vi "MPPTracker.vi"(0 "VMPP (V)":sgl, 1 "Device Code":i32=21, 2 "ID":i32=1, 3 "Channel":u8(ring) items=["1", "2", "3", "4", "5", "6", "7", "8", "9", "10", "11", "12", "13", "14", "15", "16"], 4 "instance":i32, 5 "JV after\nevery (min)":dbl=15.0 caption="Time Target (s)", 7 "Step (V)":sgl=0.01, 8 "device area (cm2)":dbl=0.16 caption="Time Target (s)", 9 "time to check (s)":sgl=10.0, 11 "error in (no error)":errorcluster, 12 "start time":timestamp, 13 "Average over":i32, 14 "AgingFile":path=path "C:/EC-Lab Development Package/Examples/Labview/V12/DefaultAging") -> (15 "error out":errorcluster)   [LabVIEW 2020]
uses:
  base_xml.llb/Type Descriptor Enumeration__ogtk.ctl
  ActiveArray.vi
  <vilib>/Utility/file.llb/Write Delimited Spreadsheet (DBL).vi
  IntensityTemperature.vi
panel:
  out "MPP start time":timestamp
  out "Time has Elapsed":bool
  out "Data 100":dbl[][](array[numeric]) format="%.2f"
  out "finished":bool
  out "XY Graph 2":cluster{"Data 101":sgl[], "Data 101":dbl[]}(graph) caption="XY Graph"
  out "Number\nof points":i32=255
  in  "Current measurement":enum16{"P(t)", "Ewe(t)", "I(t)"}(ring) caption="Draw"
  out "time (s)":sgl
  out "V (V)":sgl
  out "J (mA/cm2)":sgl
  out "P (mW/cm2)":sgl
  out "Aging Data":sgl[][](array[numeric])
  out "<P> mW/cm2":sgl=0.01
  out "last time":i32
  in  "stop 4":bool
  in  "Average last %":dbl(slide)=25.25252525252525
  in  "starting time offset (h)":dbl
  out "CAData":sgl[][](array[numeric])=[[0.0, -0.00011507986, 2.9229916e-06, 1.0], [0.010008001, -0.00048330438, 2.9229916e-06, 1.0], [0.020016002, -0.00048330438, 2.9229916e-06, 1.0], [0.030024001, -0.0007121685, 6.7342776e-06, 1.0], [0.040032003, -0.0007121685, 3.6852487e-06, 1.0], [0.050040003, -0.00063588045, 6.362202e-07, 1.0], [0.060048003, -0.00048330438, 5.2097635e-06, 1.0], [0.070056, -0.0004070163, 2.1607345e-06, 1.0], [0.080064006, -0.00017815214, 3.6852487e-06, 1.0], [0.090072006, -0.0004070163, 3.6852487e-06, 1.0], [0.100080006, -0.0004070163, 2.1607345e-06, 1.0], [0.110088006, -0.00063588045, 2.9229916e-06, 1.0], [0.120096005, -0.0005595924, 2.9229916e-06, 1.0], [0.130104, -0.0007121685, 5.2097635e-06, 1.0], [0.140112, -0.00033072825, 5.2097635e-06, 1.0], [0.15012, -0.00063588045, 2.9229916e-06, 1.0], [0.16012801, -0.0007884566, 1.3984774e-06, 1.0], [0.170136, -0.0004070163, 5.2097635e-06, 1.0], [0.18014401, -0.00063588045, 3.6852487e-06, 1.0], [0.190152, -0.00063588045, 5.97202e-06, 1.0], [0.20016001, -0.0007121685, 5.2097635e-06, 1.0], [0.210168, -0.00033072825, 2.9229916e-06, 1.0], [0.22017601, -0.0007121685, 1.3984774e-06, 1.0], [0.230184, -0.00063588045, 5.97202e-06, 1.0], [0.24019201, -0.0007884566, 5.97202e-06, 1.0], [0.2502, -0.00063588045, 4.447506e-06, 1.0], [0.260208, -0.00063588045, 4.447506e-06, 1.0], [0.27021602, -0.0007884566, 3.6852487e-06, 1.0], [0.280224, -0.00025444018, 2.9229916e-06, 1.0], [0.290232, -0.00063588045, 4.447506e-06, 1.0], [0.30024, -0.0007884566, 5.2097635e-06, 1.0], [0.31024802, -0.00048330438, 2.9229916e-06, 1.0], [0.32025602, -0.00063588045, 2.1607345e-06, 1.0], [0.330264, -0.00063588045, 3.6852487e-06, 1.0], [0.340272, -0.00063588045, 2.9229916e-06, 1.0], [0.35028002, -0.00017815214, 5.2097635e-06, 1.0], [0.36028802, -0.0007884566, 5.97202e-06, 1.0], [0.370296, -0.00063588045, 2.9229916e-06, 1.0], [0.380304, -0.00086474465, 6.7342776e-06, 1.0], [0.39031202, -0.0004070163, 2.9229916e-06, 1.0], [0.40032002, -0.0007884566, 6.362202e-07, 1.0], [0.410328, -0.0007121685, 2.1607345e-06, 1.0], [0.420336, -0.0007884566, 6.7342776e-06, 1.0], [0.43034402, -0.00063588045, 1.3984774e-06, 1.0], [0.44035202, -0.00063588045, 2.9229916e-06, 1.0], [0.45036003, -0.00063588045, 2.1607345e-06, 1.0], [0.460368, -0.00048330438, 4.447506e-06, 1.0], [0.470376, -0.00048330438, 4.447506e-06, 1.0], [0.48038402, -0.0004070163, 2.9229916e-06, 1.0], [0.49039203, -0.00033072825, 5.2097635e-06, 1.0], [0.5004, -0.00048330438, 5.2097635e-06, 1.0], [0.51040804, -0.0005595924, 5.2097635e-06, 1.0], [0.520416, -0.0005595924, 5.97202e-06, 1.0], [0.530424, -0.0007121685, 5.2097635e-06, 1.0], [0.54043204, -0.0004070163, 2.9229916e-06, 1.0], [0.55044, -0.00025444018, 5.2097635e-06, 1.0], [0.560448, -0.00048330438, 2.9229916e-06, 1.0], [0.570456, -0.0004070163, 4.447506e-06, 1.0], [0.580464, -0.0004070163, 2.9229916e-06, 1.0], [0.59047204, -0.00063588045, 2.1607345e-06, 1.0], [0.60048, -0.0007884566, 2.1607345e-06, 1.0], [0.610488, -0.00048330438, 5.2097635e-06, 1.0], [0.62049603, -0.0004070163, 2.9229916e-06, 1.0], [0.630504, -0.0007884566, 3.6852487e-06, 1.0], [0.64051205, -0.0007884566, 2.9229916e-06, 1.0], [0.65052, -0.0005595924, 5.97202e-06, 1.0], [0.660528, -0.00048330438, 2.9229916e-06, 1.0], [0.67053604, -0.00063588045, 4.447506e-06, 1.0], [0.680544, -0.00086474465, 4.447506e-06, 1.0], [0.690552, -0.00063588045, 3.6852487e-06, 1.0], [0.70056003, -0.00063588045, 1.3984774e-06, 1.0], [0.710568, -0.0005595924, 4.447506e-06, 1.0], [0.72057605, -0.00048330438, 2.9229916e-06, 1.0], [0.730584, -0.00048330438, 3.6852487e-06, 1.0], [0.740592, -0.0007884566, 4.447506e-06, 1.0], [0.75060004, -0.0005595924, 3.6852487e-06, 1.0], [0.760608, -0.0005595924, 2.9229916e-06, 1.0], [0.77061605, -0.0007884566, 4.447506e-06, 1.0], [0.78062403, -0.0010173208, 2.1607345e-06, 1.0], [0.790632, -0.00063588045, 2.1607345e-06, 1.0], [0.80064005, -0.00025444018, 2.9229916e-06, 1.0], [0.810648, -0.0005595924, 3.6852487e-06, 1.0], [0.820656, -0.00017815214, 3.6852487e-06, 1.0], [0.83066404, -0.0005595924, 4.447506e-06, 1.0], [0.840672, -0.0005595924, 1.3984774e-06, 1.0], [0.85068005, -0.00063588045, 5.2097635e-06, 1.0], [0.86068803, -0.0007884566, 5.97202e-06, 1.0], [0.870696, -0.0004070163, 4.447506e-06, 1.0], [0.88070405, -0.00033072825, 4.447506e-06, 1.0], [0.890712, -0.0005595924, 3.6852487e-06, 1.0], [0.90072006, -0.0005595924, 4.447506e-06, 1.0], [0.91072804, -0.0007121685, 4.447506e-06, 1.0], [0.920736, -0.00063588045, 2.1607345e-06, 1.0], [0.93074405, -0.0005595924, 5.2097635e-06, 1.0], [0.940752, -0.0004070163, 2.1607345e-06, 1.0], [0.95076, -0.0004070163, 2.1607345e-06, 1.0], [0.96076804, -0.00025444018, 2.9229916e-06, 1.0], [0.970776, -0.00063588045, 3.6852487e-06, 1.0], [0.98078406, -0.00063588045, 2.9229916e-06, 1.0], [0.99079204, 0.0001270001, 2.1607345e-06, 1.0], [1.0008, 0.09945406, 5.5518736e-05, 1.0], [1.010808, 0.09960663, 2.3503935e-05, 1.0], [1.0208161, 0.09945406, 2.2741679e-05, 1.0], [1.0308241, 0.099759206, 2.5790707e-05, 1.0], [1.040832, 0.09930148, 2.4266194e-05, 1.0], [1.05084, 0.099377766, 2.1217164e-05, 1.0], [1.060848, 0.09945406, 2.2741679e-05, 1.0], [1.0708561, 0.09953035, 2.1217164e-05, 1.0], [1.0808641, 0.09953035, 2.3503935e-05, 1.0], [1.090872, 0.09953035, 2.3503935e-05, 1.0], [1.10088, 0.09968292, 2.4266194e-05, 1.0], [1.110888, 0.09945406, 2.4266194e-05, 1.0], [1.120896, 0.09953035, 2.6552963e-05, 1.0], [1.1309041, 0.099377766, 2.6552963e-05, 1.0], [1.140912, 0.09953035, 2.502845e-05, 1.0], [1.15092, 0.09922519, 2.1217164e-05, 1.0], [1.160928, 0.09953035, 2.3503935e-05, 1.0], [1.170936, 0.099377766, 1.969265e-05, 1.0], [1.1809441, 0.09930148, 2.4266194e-05, 1.0], [1.1909521, 0.09953035, 2.4266194e-05, 1.0], [1.20096, 0.09953035, 2.3503935e-05, 1.0], [1.210968, 0.09953035, 2.4266194e-05, 1.0], [1.220976, 0.09968292, 2.2741679e-05, 1.0], [1.2309841, 0.09960663, 2.4266194e-05, 1.0], [1.2409921, 0.0998355, 2.4266194e-05, 1.0], [1.251, 0.09945406, 2.1217164e-05, 1.0], [1.261008, 0.09968292, 2.502845e-05, 1.0], [1.271016, 0.09930148, 2.4266194e-05, 1.0], [1.2810241, 0.09968292, 1.8930392e-05, 1.0], [1.2910321, 0.09930148, 2.4266194e-05, 1.0], [1.30104, 0.09930148, 2.5790707e-05, 1.0], [1.311048, 0.09907261, 2.4266194e-05, 1.0], [1.321056, 0.09945406, 2.1217164e-05, 1.0], [1.3310641, 0.09968292, 2.5790707e-05, 1.0], [1.3410721, 0.09914891, 2.1979422e-05, 1.0], [1.3510801, 0.09945406, 2.502845e-05, 1.0], [1.361088, 0.09945406, 2.5790707e-05, 1.0], [1.371096, 0.09960663, 2.1217164e-05, 1.0], [1.381104, 0.09930148, 2.4266194e-05, 1.0], [1.3911121, 0.09930148, 2.4266194e-05, 1.0], [1.4011201, 0.09998807, 2.4266194e-05, 1.0], [1.411128, 0.09968292, 2.4266194e-05, 1.0], [1.421136, 0.09960663, 2.1217164e-05, 1.0], [1.431144, 0.09998807, 2.3503935e-05, 1.0], [1.4411521, 0.09968292, 2.1217164e-05, 1.0], [1.4511601, 0.09953035, 2.5790707e-05, 1.0], [1.461168, 0.09960663, 2.5790707e-05, 1.0], [1.471176, 0.09968292, 2.2741679e-05, 1.0], [1.481184, 0.09930148, 2.4266194e-05, 1.0], [1.4911921, 0.09945406, 2.2741679e-05, 1.0], [1.5012001, 0.09960663, 2.0454907e-05, 1.0], [1.511208, 0.09945406, 2.3503935e-05, 1.0], [1.521216, 0.099377766, 1.969265e-05, 1.0], [1.531224, 0.09930148, 2.1217164e-05, 1.0], [1.5412321, 0.09914891, 2.2741679e-05, 1.0], [1.5512401, 0.09953035, 2.2741679e-05, 1.0], [1.5612481, 0.099377766, 2.2741679e-05, 1.0], [1.571256, 0.099377766, 2.5790707e-05, 1.0], [1.581264, 0.099759206, 2.4266194e-05, 1.0], [1.5912721, 0.09968292, 2.2741679e-05, 1.0], [1.6012801, 0.09930148, 2.4266194e-05, 1.0], [1.6112881, 0.09930148, 2.4266194e-05, 1.0], [1.621296, 0.09960663, 2.1217164e-05, 1.0], [1.631304, 0.09968292, 2.5790707e-05, 1.0], [1.641312, 0.09953035, 2.5790707e-05, 1.0], [1.6513201, 0.09930148, 2.502845e-05, 1.0], [1.6613281, 0.09945406, 2.4266194e-05, 1.0], [1.671336, 0.09953035, 2.1217164e-05, 1.0], [1.681344, 0.099377766, 2.4266194e-05, 1.0], [1.691352, 0.09960663, 2.2741679e-05, 1.0], [1.7013601, 0.09968292, 2.3503935e-05, 1.0], [1.7113681, 0.09907261, 2.5790707e-05, 1.0], [1.7213761, 0.09953035, 2.4266194e-05, 1.0], [1.731384, 0.099377766, 2.2741679e-05, 1.0], [1.741392, 0.09960663, 2.502845e-05, 1.0], [1.7514001, 0.09953035, 2.502845e-05, 1.0], [1.7614081, 0.09945406, 2.6552963e-05, 1.0], [1.7714161, 0.099377766, 2.502845e-05, 1.0], [1.781424, 0.09960663, 2.5790707e-05, 1.0], [1.791432, 0.09907261, 2.502845e-05, 1.0], [1.8014401, 0.09930148, 2.0454907e-05, 1.0], [1.8114481, 0.09968292, 2.1979422e-05, 1.0], [1.8214561, 0.09930148, 2.2741679e-05, 1.0], [1.831464, 0.09930148, 2.4266194e-05, 1.0], [1.841472, 0.09914891, 2.0454907e-05, 1.0], [1.85148, 0.099377766, 2.2741679e-05, 1.0], [1.8614881, 0.09953035, 2.502845e-05, 1.0], [1.8714961, 0.09945406, 2.3503935e-05, 1.0], [1.881504, 0.09907261, 2.502845e-05, 1.0], [1.891512, 0.099377766, 2.2741679e-05, 1.0], [1.90152, 0.09945406, 2.5790707e-05, 1.0], [1.9115281, 0.09953035, 2.5790707e-05, 1.0], [1.9215361, 0.099759206, 2.4266194e-05, 1.0], [1.9315441, 0.09945406, 2.6552963e-05, 1.0], [1.941552, 0.09945406, 2.0454907e-05, 1.0], [1.95156, 0.09945406, 2.5790707e-05, 1.0], [1.9615681, 0.09991179, 2.5790707e-05, 1.0], [1.9715761, 0.09945406, 2.3503935e-05, 1.0], [1.9815841, 0.09930148, 2.3503935e-05, 1.0], [1.991592, 0.09960663, 2.5790707e-05, 1.0], [2.0016, 0.19969657, 6.3903564e-05, 1.0], [2.0116081, 0.19939142, 4.256037e-05, 1.0], [2.021616, 0.19931513, 4.408488e-05, 1.0], [2.031624, 0.1994677, 4.332262e-05, 1.0], [2.0416322, 0.199544, 4.332262e-05, 1.0], [2.05164, 0.1994677, 4.4847136e-05, 1.0], [2.0616481, 0.19962028, 4.332262e-05, 1.0], [2.071656, 0.19977286, 4.332262e-05, 1.0], [2.081664, 0.19992544, 4.256037e-05, 1.0], [2.0916722, 0.19977286, 4.4847136e-05, 1.0], [2.10168, 0.19977286, 4.408488e-05, 1.0], [2.1116881, 0.20007801, 4.4847136e-05, 1.0], [2.121696, 0.19992544, 4.103585e-05, 1.0], [2.131704, 0.199544, 4.256037e-05, 1.0], [2.1417122, 0.199544, 4.6371653e-05, 1.0], [2.15172, 0.19969657, 4.256037e-05, 1.0], [2.1617281, 0.199544, 4.256037e-05, 1.0], [2.171736, 0.19984914, 4.256037e-05, 1.0], [2.181744, 0.1994677, 4.256037e-05, 1.0], [2.1917522, 0.20000172, 4.256037e-05, 1.0], [2.20176, 0.199544, 4.6371653e-05, 1.0], [2.2117682, 0.1994677, 4.0273593e-05, 1.0], [2.221776, 0.19969657, 4.332262e-05, 1.0], [2.231784, 0.19962028, 4.332262e-05, 1.0], [2.241792, 0.199544, 4.408488e-05, 1.0], [2.2518, 0.19977286, 4.332262e-05, 1.0], [2.2618082, 0.1994677, 4.408488e-05, 1.0], [2.271816, 0.19969657, 4.6371653e-05, 1.0], [2.281824, 0.19969657, 4.408488e-05, 1.0], [2.291832, 0.1994677, 4.332262e-05, 1.0], [2.30184, 0.19984914, 4.408488e-05, 1.0], [2.3118482, 0.19923884, 3.9511335e-05, 1.0], [2.321856, 0.19962028, 4.256037e-05, 1.0], [2.331864, 0.19969657, 4.1798106e-05, 1.0], [2.341872, 0.19969657, 4.6371653e-05, 1.0], [2.35188, 0.19969657, 4.4847136e-05, 1.0], [2.3618882, 0.19969657, 4.6371653e-05, 1.0], [2.371896, 0.19939142, 4.103585e-05, 1.0], [2.3819041, 0.19939142, 4.332262e-05, 1.0], [2.391912, 0.1994677, 4.103585e-05, 1.0], [2.40192, 0.19962028, 4.1798106e-05, 1.0], [2.4119282, 0.19962028, 4.4847136e-05, 1.0], [2.421936, 0.1994677, 4.332262e-05, 1.0], [2.4319441, 0.19977286, 4.408488e-05, 1.0], [2.441952, 0.20007801, 4.408488e-05, 1.0], [2.45196, 0.19984914, 4.5609395e-05, 1.0], [2.4619682, 0.19962028, 4.256037e-05, 1.0], [2.471976, 0.19984914, 4.4847136e-05, 1.0], [2.4819841, 0.19939142, 4.6371653e-05, 1.0], [2.491992, 0.199544, 4.1798106e-05, 1.0], [2.502, 0.19984914, 4.408488e-05, 1.0], [2.5120082, 0.19931513, 4.332262e-05, 1.0], [2.522016, 0.199544, 4.6371653e-05, 1.0], [2.5320241, 0.199544, 4.4847136e-05, 1.0], [2.542032, 0.19931513, 4.408488e-05, 1.0]] format="%.2f"
  in  "CA Parameters":T1={"tb"=0.0001, "Steps"=[{"vs_initial"=TRUE, "Voltage_step"=0.0, "Duration_step"=1.0}, {"vs_initial"=TRUE, "Voltage_step"=0.1, "Duration_step"=1.0}, {"vs_initial"=TRUE, "Voltage_step"=0.2, "Duration_step"=1.0}], "Step_number"=1, "N_Cycles"=0, "Record_every_dI"=10.0, "Record_every_dT"=0.1, "I_Range"=12, "E_Range"=0, "Bandwidth"=5, "em"=1, "ce"=0} {"tb" min=2.5e-05 max=1 format="%^_3e"; "ce" items=["Standard", "CE to ground"]; "N_Cycles" min=0 max=1000000; "Step_number" min=0 max=99; "E_Range" items=["±2.5V", "±5V", "±10V", "Auto"]; "Bandwidth" items=["1"=1, "2"=2, "3"=3, "4"=4, "5"=5, "6"=6, "7"=7, "8"=8, "9"=9]; "Record_every_dT" min=0.0001 max=1000 format="%^_3e"; "Record_every_dI" format="%^_3e"; "I_Range" items=["1pA", "1nA", "10nA", "100nA", "1µA", "10µA", "100µA", "1mA", "10mA", "100mA", "1A", "Booster", "Auto"]; "Steps"."Duration_step" min=0.001 max=80000 format="%^_3e"; "Steps"."Voltage_step" min=-10 max=10 format="%^_3e"}
  # "Connection *"
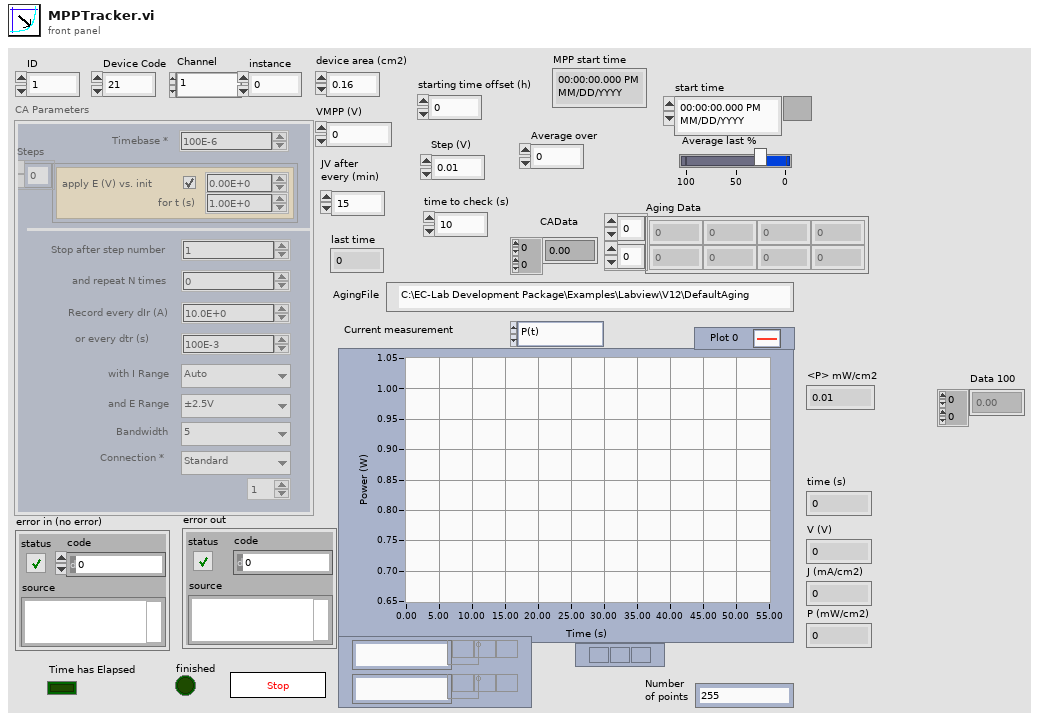
[diagram p1: front panel]
types:
  T1 = cluster{"tb":sgl, "Steps":cluster{"vs_initial":bool, "Voltage_step":sgl, "Duration_step":sgl}[], "Step_number":i32, "N_Cycles":i32, "Record_every_dI":sgl, "Record_every_dT":sgl, "I_Range":u16, "E_Range":u16, "Bandwidth":u16, "em":u16, "ce":u16}
  T2 = typedef "Type Descriptor Enumeration__ogtk.ctl" = enum8{"<Null>", "I8", "I16", "I32", "I64", "U8", "U16", "U32", "U64", "SGL", "DBL", "EXT", "CSG", "CDB", "CXT", "0x0F", "0x10", "0x11", "0x12", "0x13", "0x14", "Enum U8", "Enum U16", "Enum U32", "Enum U64", "SGL PQ", "DBL PQ", "EXT PQ", "CSG PQ", "CDB PQ", "CXT PQ", "0x1F", "0x20", "Boolean", "0x22", "0x23", "0x24", "0x25", "0x26", "0x27", "0x28", "0x29", "0x2A", "0x2B", "0x2C", "0x2D", "0x2E", "0x2F", "String", "0x31", "Path", "Pict", "0x34", "0x35", "0x36", "DAQ", "0x38", "0x39", "0x3A", "0x3B", "0x3C", "0x3D", "0x3E", "0x3F", "Array", "0x41", "0x42", "0x43", "0x44", "0x45", "0x46", "0x47", "0x48", "0x49", "0x4A", "0x4B", "0x4C", "0x4D", "0x4E", "0x4F", "Cluster", "0x51", "0x52", "Variant", "Waveform", "0x55", "0x56", "0x57", "0x58", "0x59", "0x5A", "0x5B", "0x5C", "0x5D", "0x5E", "0x5F", "0x60", "0x61", "0x62", "0x63", "0x64", "0x65", "0x66", "0x67", "0x68", "0x69", "0x6A", "0x6B", "0x6C", "0x6D", "0x6E", "0x6F", "Refnum"}
  T3 = cluster{"Data Type":T2, "Format String":string}[]
  T4 = cluster{"vs_initial":bool, "Voltage_step":sgl, "Duration_step":sgl}[]
  T5 = cluster{"vs_initial":bool, "Voltage_step":sgl, "Duration_step":sgl}
  T6 = cluster{"Label":string, "type":i32, "valeur":u32, "index":i32}[]
  T7 = cluster{"IRQskipped":i32, "NbRaws":i32, "NbCols":i32, "Technique Index":i32, "TechniqueID":i32, "PrcessIndex":i32, "loop":i32, "StartTime":dbl, "MuxPad":i32}
  T8 = cluster{"State":i32, "MemFilled":i32, "TimeBase":sgl, " Ewe":sgl, " EweRangeMin":sgl, " EweRangeMax":sgl, "Ece":sgl, "EceRangeMin":sgl, "EceRangeMax":sgl, "Eoverflow":i32, "I":sgl, "IRange":i32, "Ioverflow":i32, "ElapsedTime":sgl, "Freq":sgl, "Rcomp":sgl, "Saturation":sgl, "OptErr":i32, "OptPos":i32}
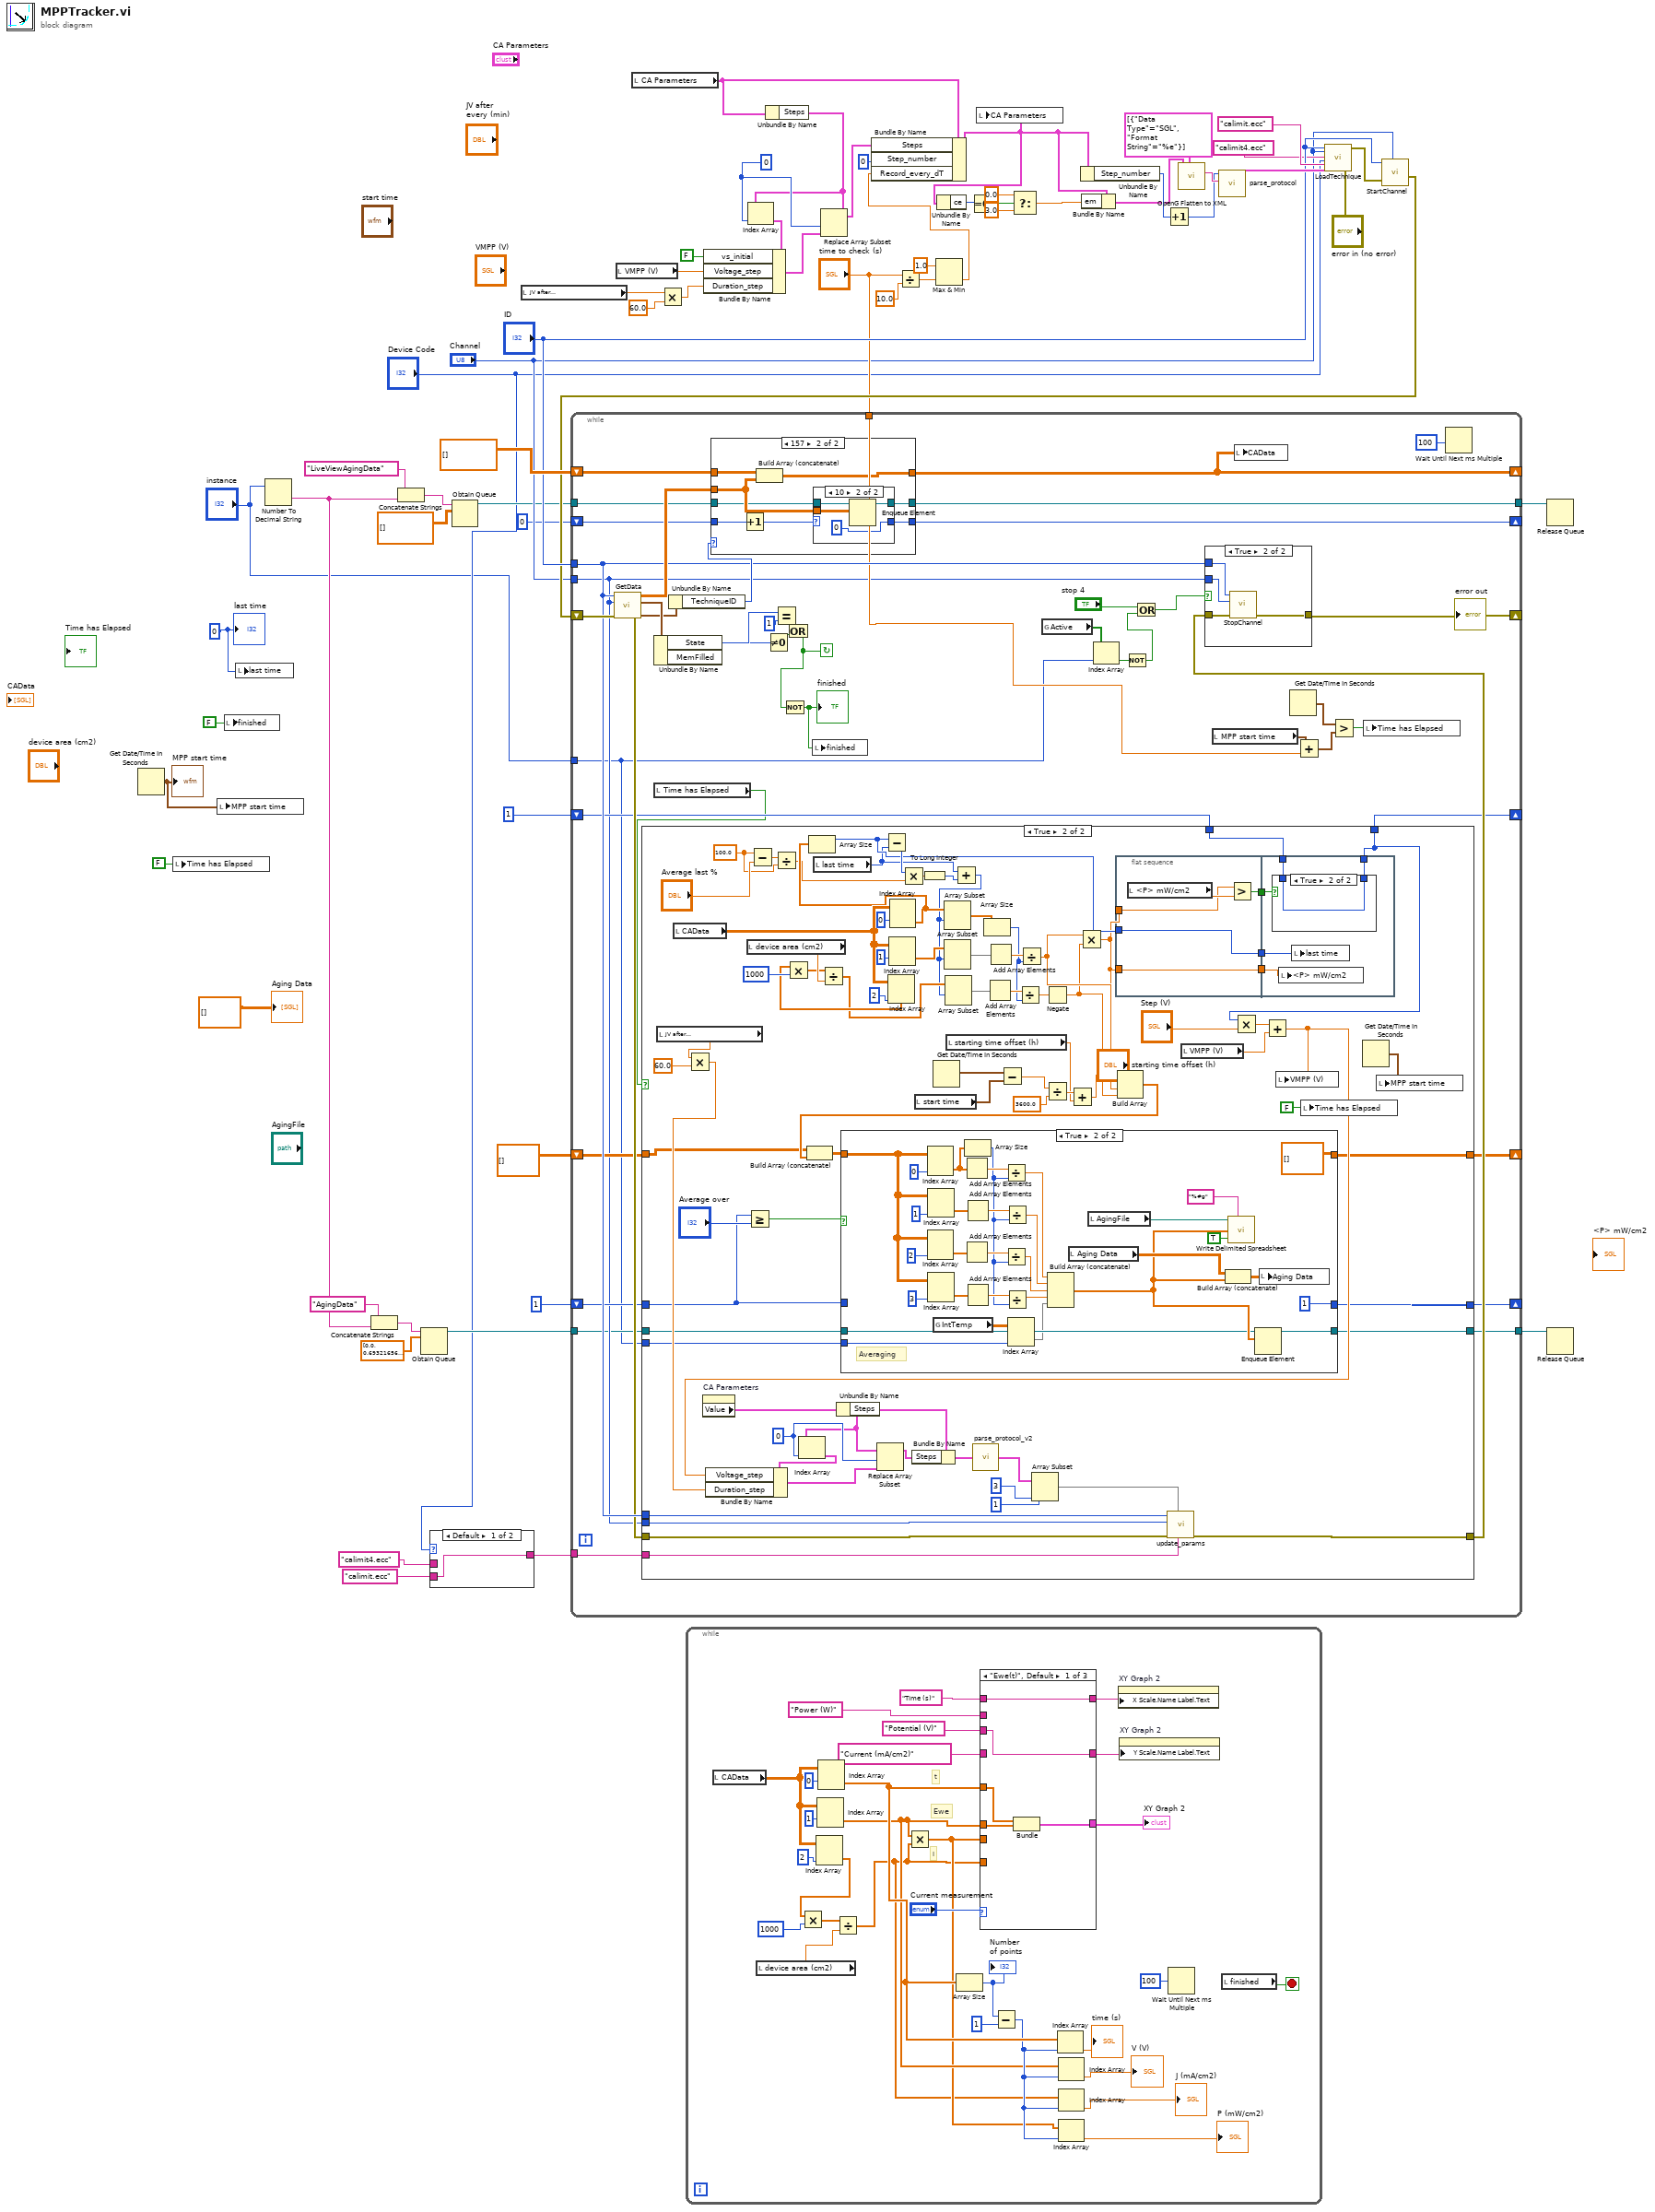
[diagram p0: block diagram]
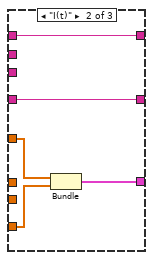
[diagram p3: hidden frame]
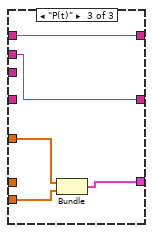
[diagram p4: hidden frame]
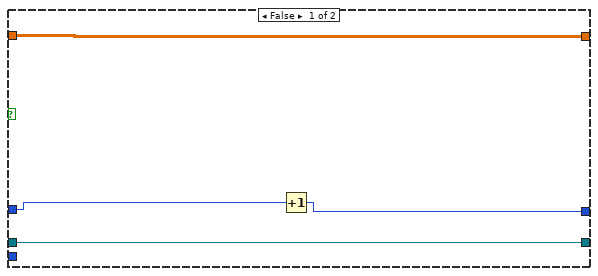
[diagram p6: hidden frame]
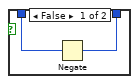
[diagram p7: hidden frame]
diagram:
  w30 = 0 ("last time")
  w50 = 0 ("index")
  n1 = Get Date/Time In Seconds() -> (seconds since 1Jan1904=w19:timestamp)
  "MPP start time" <- w19
  n2 = local write "Time has Elapsed"(FALSE ("Time has Elapsed")) -> ()
  n3 = local write "MPP start time"(w19) -> ()
  n4 = local write "finished"(FALSE ("finished")) -> ()
  n5 = local write "last time"(w30) -> ()
  n6 = Number To Decimal String(number="instance") -> (decimal integer string=w9:string)  [unwired: 1 in]
  n7 = Concatenate Strings("AgingData" ("name (unnamed)"), w9) -> (w11:string)
  n8 = Concatenate Strings("LiveViewAgingData" ("name (unnamed)"), w9) -> (w17:string)
  n9 = Obtain Queue(name (unnamed)=w11, element data type=dbl[] [0.0, 0.6932165634222212, 0.002936372303467471, 0.2869923716049554, 0.0005841850023007069, 0.39914193749427795, 0.001463602161096093, 0.0, 0.0, 0.0, 0.0, 0.0, 0.0, inf] ("appended array 2")) -> (queue out=w8:refnum<queue>)  [unwired: 3 in, 2 out]
  n10 = case shown="Default" "Device Code" {
    tunnel: "calimit.ecc" ("FName") -> [w64 _]
    tunnel: [w64 w65] -> w3
    tunnel: "calimit4.ecc" ("FName") -> [_ w65]
    frame Default {
    }
    frame 12, 16, 20, 21, 23, 27 {
    }
  }
  n11 = Obtain Queue(name (unnamed)=w17, element data type=sgl[][] []) -> (queue out=w14:refnum<queue>)  [unwired: 3 in, 2 out]
  n12 = local read "JV after\nevery (min)"() -> (w43:dbl)
  n13 = local read "VMPP (V)"() -> (w46:sgl)
  n14 = local read "CA Parameters"() -> (w45:T1)
  n15 = Multiply(x=w43, y=60.0) -> (x*y=w42:dbl)
  n16 = while {
    stop <- w93 stop-if-true
    # "I"
    # "Ewe"
    # "t"
    n17 = local read "CAData"() -> (w83:sgl[][])
    n18 = local read "device area (cm2)"() -> (w69:dbl)
    n19 = Index Array(array=w83, index (col)=2 ("indice désactivé (col)")) -> (element=w67:sgl[])  [unwired: 1 in]
    n20 = Multiply(x=w67, y=1000) -> (x*y=w70:sgl[])
    n21 = Index Array(array=w83, index (col)=1 ("Index")) -> (element=w76:sgl[])  [unwired: 1 in]
    n22 = Index Array(array=w83, index (col)=0 ("Index")) -> (element=w78:sgl[])  [unwired: 1 in]
    n23 = Divide(x=w70, y=w69) -> (x/y=w66:dbl[])
    n24 = Multiply(x=w76, y=w66) -> (x*y=w75:dbl[])
    n25 = Array Size(array=w78) -> (size(s)=w80:i32)
    "Number\nof points" <- w80
    n26 = case shown="\"Ewe(t)\", Default" "Current measurement" {
      tunnel: w78 -> [w99 w100 w107]
      tunnel: [w96 w101 w105] -> w82
      tunnel: "Potential (V)" ("Y Scale.Name Label.Text") -> [w98 _ _]
      tunnel: "Current (mA/cm2)" ("Y Scale.Name Label.Text") -> [_ w104 _]
      tunnel: [w98 w104 w108] -> w87
      tunnel: [w97 w103 w109] -> w86
      tunnel: "Time (s)" ("Y Scale.Name Label.Text") -> [w97 w103 w109]
      tunnel: w76 -> [w95 _ _]
      tunnel: w66 -> [_ w102 _]
      tunnel: "Power (W)" ("Y Scale.Name Label.Text") -> [_ _ w108]
      tunnel: w75 -> [_ _ w106]
      frame "Ewe(t)", Default {
        n27 = Bundle("CAData"=w99, "CAData"=w95) -> (w96:cluster{"CAData":sgl[], "CAData":sgl[]})  [unwired: 1 in]
      }
      frame "I(t)" {
        n28 = Bundle("CAData"=w100, w102) -> (w101:cluster{"CAData":sgl[], dbl[]})  [unwired: 1 in]
      }
      frame "P(t)" {
        n29 = Bundle("CAData"=w107, w106) -> (w105:cluster{"CAData":sgl[], dbl[]})  [unwired: 1 in]
      }
    }
    "XY Graph 2" <- w82
    n30 = Subtract(x=w80, y=1) -> (x-y=w77:i32)
    n31 = Index Array(array=w78, index=w77) -> (element=→"time (s)":sgl)
    n32 = Index Array(array=w76, index=w77) -> (element=→"V (V)":sgl)
    n33 = Index Array(array=w66, index=w77) -> (element=→"J (mA/cm2)":dbl)
    n34 = Index Array(array=w75, index=w77) -> (element=→"P (mW/cm2)":dbl)
    n35 = property on="XY Graph 2" class="XYGraph (strict)"("X Scale.Name Label.Text"=w86) -> ()  [unwired: 2 in, 2 out]
    n36 = property on="XY Graph 2" class="XYGraph (strict)"("Y Scale.Name Label.Text"=w87) -> ()  [unwired: 2 in, 2 out]
    n37 = Wait Until Next ms Multiple(millisecond multiple=u32 100) -> ()  [unwired: 1 out]
    n38 = local read "finished"() -> (w93:bool)
  }
  n39 = Unbundle By Name(w45) -> ("Steps"=w49:T4)
  n40 = Index Array(array=w49, index=w50) -> (element=w48:T5)
  n41 = Bundle By Name(cluster=w48, "vs_initial"=FALSE, "Voltage_step"=w46, "Duration_step"=w42) -> (w51:T5)
  n42 = Replace Array Subset(array=w49, new element=w51, index=w50) -> (w44:T4)
  n43 = Divide(x="time to check (s)", y=sgl 10.0) -> (x/y=w25:sgl)
  n44 = Max & Min(x=1.0, y=w25) -> (min(x,y)=w26:dbl)  [unwired: 1 out]
  n45 = Bundle By Name(cluster=w45, "Steps"=w44, "Step_number"=0, "Record_every_dT"=w26) -> (w40:T1)
  n46 = Unbundle By Name(w40) -> ("ce"=w54:u16)
  n47 = Equal To 0?(x=w54) -> (x = 0?=w53:bool)
  n48 = local write "CA Parameters"(w40) -> ()
  n49 = Select(t=0.0, s=w53, f=3.0) -> (s? t:f=w57:dbl)
  n50 = Unbundle By Name(w40) -> ("Step_number"=w59:i32)
  n51 = Bundle By Name(cluster=w40, "em"=w57) -> (w52:T1)
  n52 = Increment(x=w59) -> (x+1=w58:i32)
  n53 = call "OpenG Flatten to XML.vi"("Type Formats (default)"=T3 [{"Data Type"=enum."SGL", "Format String"="%e"}] ("Type Formats"), "LabVIEW Data"=w52) -> ("XML String"=w62:string)  [unwired: 8 in, 1 out]
  n54 = call "parse_protocol.vi"("XML String In"=w62, "index array"=w58) -> ("Params Values"=w61:T6)  [unwired: 7 in]
  n55 = call "LoadTechnique.vi"("ID"="ID", "Selected Channel"="Channel", "FName4"="calimit4.ecc" ("FName"), "Device Code"="Device Code", "FName"="calimit.ecc", "Protocol Parameters"=w61, "error in (no error)"="error in (no error)") -> ("error out"=w63:errorcluster)  [unwired: 12 in]
  n56 = call "StartChannel.vi"("error in (no error)"=w63, "Channel"="Channel", "ID"="ID") -> ("error out"=w34:errorcluster)  [unwired: 8 in]
  n57 = while {
    shift-right: [w149] -> w31
    shift-left: w34 -> [w151]
    shift-right: [w125] -> _
    shift-left: sgl[][] [] -> [w147]
    tunnel: "Channel" -> [w117]
    tunnel: "ID" -> [w141]
    tunnel: w3 -> [w138]
    shift-right: [w137] -> _
    shift-left: 1 -> [w136]
    tunnel: "time to check (s)" -> [w121]
    shift-right: [w128] -> _
    shift-left: 1 -> [w124]
    shift-right: [w127] -> _
    shift-left: dbl[][] [] -> [w126]
    tunnel: w14 -> [w116]
    tunnel: [w115] -> w13
    tunnel: w8 -> [w114]
    tunnel: [w113] -> w7
    tunnel: "instance" -> [w112]
    shift-right: [w110] -> _
    shift-left: 0 -> [w111]
    stop <- w135 continue-if-true
    n58 = call "GetData.vi"("error in (no error)"=w151, "Channel"=w117, "ID"=w141) -> ("error out"=w140:errorcluster, "Data information"=w143:T7, "Current values"=w146:T8, "Data"=w148:dbl[][])  [unwired: 5 in]
    n59 = Unbundle By Name(w146) -> ("State"=w145:i32, "MemFilled"=w144:i32)
    n60 = local read "Time has Elapsed"() -> (w123:bool)
    n61 = case shown="True" w123 {
      tunnel: w140 -> [w159 w238]
      tunnel: [w159 w237] -> w139
      tunnel: w141 -> [_ w196]
      tunnel: w117 -> [_ w172]
      tunnel: w138 -> [_ w235]
      tunnel: [w158 w189] -> w137
      tunnel: w136 -> [w158 w190]
      tunnel: w124 -> [w157 w174]
      tunnel: [w157 w175] -> w128
      tunnel: w126 -> [w156 w166]
      tunnel: [w156 w173] -> w127
      tunnel: w114 -> [w155 w162]
      tunnel: [w155 w161] -> w113
      tunnel: w112 -> [_ w160]
      frame False {
      }
      frame True {
        w215 = 100.0 ("x")
        w233 = 0 ("index")
        n62 = local read "JV after\nevery (min)"() -> (w179:dbl)
        n63 = local read "CAData"() -> (w229:sgl[][])
        n64 = Multiply(x=w179, y=60.0) -> (x*y=w180:dbl)
        n65 = property on="CA Parameters" class="Clust (strict)"() -> ("Value"=w178:T1)  [unwired: 2 in, 2 out]
        n66 = local read "device area (cm2)"() -> (w222:dbl)
        n67 = Greater Or Equal?(x=w174, y="Average over") -> (x >= y?=w177:bool)
        n68 = Subtract(x=w215, y="Average last %") -> (x-y=w216:dbl)
        n69 = Divide(x=w216, y=w215) -> (x/y=w213:dbl)
        n70 = local read "last time"() -> (w184:i32)
        n71 = Unbundle By Name(w178) -> ("Steps"=w232:T4)
        n72 = Index Array(array=w232, index=w233) -> (element=w195:T5)
        n73 = Index Array(array=w229, index (col)=2 ("indice désactivé (col)")) -> (element=w205:sgl[])  [unwired: 1 in]
        n74 = Multiply(x=w205, y=1000) -> (x*y=w221:sgl[])
        n75 = Divide(x=w221, y=w222) -> (x/y=w204:dbl[])
        n76 = Index Array(array=w229, index (col)=1 ("Index")) -> (element=w219:sgl[])  [unwired: 1 in]
        n77 = Index Array(array=w229, index (col)=0 ("Index")) -> (element=w218:sgl[])  [unwired: 1 in]
        n78 = Array Size(array=w218) -> (size(s)=w187:i32)
        n79 = Subtract(x=w187, y=w184) -> (x-y=w214:i32)
        n80 = Multiply(x=w214, y=w213) -> (x*y=w212:dbl)
        n81 = local read "start time"() -> (w225:timestamp)
        n82 = To Long Integer(number=w212) -> (32bit integer=w183:i32)
        n83 = Get Date/Time In Seconds() -> (seconds since 1Jan1904=w224:timestamp)
        n84 = local read "starting time offset (h)"() -> (w168:dbl)
        n85 = Add(x=w184, y=w183) -> (x+y=w182:i32)
        n86 = Array Subset(array=w218, index=w182) -> (w211:sgl[])  [unwired: 1 in]
        n87 = Array Subset(array=w219, index=w182) -> (w209:sgl[])  [unwired: 1 in]
        n88 = Array Subset(array=w204, index=w182) -> (w210:dbl[])  [unwired: 1 in]
        n89 = Array Size(array=w211) -> (size(s)=w206:i32)
        n90 = Add Array Elements(numeric array=w210) -> (sum=w207:dbl)
        n91 = Add Array Elements(numeric array=w209) -> (sum=w208:sgl)
        n92 = Subtract(x=w224, y=w225) -> (x-y=w169:dbl)
        n93 = Divide(x=w207, y=w206) -> (x/y=w203:dbl)
        n94 = Divide(x=w208, y=w206) -> (x/y=w202:sgl)
        n95 = Negate(x=w203) -> (-x=w201:dbl)
        n96 = Divide(x=w169, y=3600.0) -> (x/y=w170:dbl)
        n97 = Add(x=w170, y=w168) -> (x+y=w220:dbl)
        n98 = Multiply(x=w202, y=w201) -> (x*y=w185:dbl)
        n99 = flat-sequence {
          tunnel: [w277] -> w191
          tunnel: w185 -> [w276]
          tunnel: w185 -> [w275]
          tunnel: [w275] -> w188
          tunnel: w187 -> [w274]
          tunnel: [w274] -> w186
          tunnel: w191 -> [w283]
          tunnel: w190 -> [w282]
          tunnel: [w281] -> w189
          tunnel: w188 -> [w280]
          tunnel: w186 -> [w279]
          frame #0 {
            n100 = local read "<P> mW/cm2"() -> (w278:sgl)
            n101 = Greater?(x=w276, y=w278) -> (0:w277:bool)
          }
          frame #1 {
            n102 = case shown="True" w283 {
              tunnel: w282 -> [w285 w286]
              tunnel: [w284 w286] -> w281
              frame False {
                n103 = Negate(x=w285) -> (-x=w284:i32)
              }
              frame True {
              }
            }
            n104 = local write "<P> mW/cm2"(w280) -> ()
            n105 = local write "last time"(w279) -> ()
          }
        }
        n106 = Build Array(w220, w185, w202, w201) -> (w167:dbl[])
        n107 = Build Array (concatenate)(w166, w167) -> (w163:dbl[][])
        n108 = case shown="True" w177 {
          tunnel: w174 -> [w242 _]
          tunnel: [w241 1] -> w175
          tunnel: w163 -> [w240 w258]
          tunnel: [w240 dbl[][] []] -> w173
          tunnel: w162 -> [w239 w247]
          tunnel: [w239 w246] -> w161
          tunnel: w160 -> [_ w244]
          frame False {
            n109 = Increment(x=w242) -> (x+1=w241:i32)
          }
          frame True {
            # "Averaging"
            n110 = Index Array(array=w258, index (col)=0 ("Index")) -> (element=w265:dbl[])  [unwired: 1 in]
            n111 = Index Array(array=w258, index (col)=2 ("Index")) -> (element=w261:dbl[])  [unwired: 1 in]
            n112 = Index Array(array=w258, index (col)=1 ("Index")) -> (element=w264:dbl[])  [unwired: 1 in]
            n113 = Index Array(array=w258, index (col)=3 ("Index")) -> (element=w260:dbl[])  [unwired: 1 in]
            n114 = global read "IntensityTemperature.vi" "IntTemp"() -> (w245:dbl[][])
            n115 = Add Array Elements(numeric array=w265) -> (sum=w266:dbl)
            n116 = Add Array Elements(numeric array=w261) -> (sum=w262:dbl)
            n117 = Array Size(array=w265) -> (size(s)=w257:i32)
            n118 = Add Array Elements(numeric array=w264) -> (sum=w263:dbl)
            n119 = Add Array Elements(numeric array=w260) -> (sum=w259:dbl)
            n120 = Divide(x=w266, y=w257) -> (x/y=w256:dbl)
            n121 = Divide(x=w262, y=w257) -> (x/y=w254:dbl)
            n122 = Divide(x=w263, y=w257) -> (x/y=w255:dbl)
            n123 = Divide(x=w259, y=w257) -> (x/y=w253:dbl)
            n124 = Index Array(array=w245, index (col)=w244) -> (element=w243:dbl[])  [unwired: 1 in]
            n125 = Build Array (concatenate)(w256, w255, w254, w253, w243) -> (w248:dbl[])
            n126 = local read "Aging Data"() -> (w269:sgl[][])
            n127 = local read "AgingFile"() -> (w271:path)
            n128 = Build Array (concatenate)(w269, w248) -> (w272:dbl[][])
            n129 = call-poly <vilib>:"Write Delimited Spreadsheet.vi"("file path (dialog if empty)"=w271, "format (%.3f)"="%#g", "1D data"=w248, "append to file? (new file:F)"=TRUE ("append to file? (F)")) -> ()  [unwired: 10 in, 2 out]
            n130 = Enqueue Element(queue=w247, element=w248) -> (queue out=w246:refnum<queue>)  [unwired: 2 in, 2 out]
            n131 = local write "Aging Data"(w272) -> ()
          }
        }
        n132 = local read "VMPP (V)"() -> (w198:sgl)
        n133 = Multiply(x=w189, y="Step (V)") -> (x*y=w199:sgl)
        n134 = Add(x=w199, y=w198) -> (x+y=w197:sgl)
        n135 = Bundle By Name(cluster=w195, "Voltage_step"=w197, "Duration_step"=w180) -> (w234:T5)
        n136 = Replace Array Subset(array=w232, new element=w234, index=w233) -> (w231:T4)
        n137 = Bundle By Name(cluster=w178, "Steps"=w231) -> (w230:T1)
        n138 = call "parse_protocol_v2.vi"("Protocol Cluster"=w230) -> ("Params Values"=w194:T6)
        n139 = Array Subset(array=w194, index=1, length=3) -> (w193:T6)
        n140 = call "update_params.vi"("EccFileName"=w235, "Params"=w193, "error in (no error)"=w238, "Channel"=w172, "ID"=w196) -> ("error out"=w237:errorcluster)  [unwired: 6 in]
        n141 = local write "VMPP (V)"(w197) -> ()
        n142 = local write "Time has Elapsed"(FALSE ("Time has Elapsed")) -> ()
        n143 = Get Date/Time In Seconds() -> (seconds since 1Jan1904=w164:timestamp)
        n144 = local write "MPP start time"(w164) -> ()
      }
    }
    n145 = Unbundle By Name(w143) -> ("TechniqueID"=w142:i32)
    n146 = case shown="157" w142 {
      tunnel: w148 -> [_ w300]
      tunnel: w147 -> [w294 w302]
      tunnel: [w294 w301] -> w125
      tunnel: w116 -> [w293 w299]
      tunnel: [w293 w298] -> w115
      tunnel: w111 -> [w292 w297]
      tunnel: [w292 w295] -> w110
      frame 0, Default {
      }
      frame 157 {
        n147 = Increment(x=w297) -> (x+1=w296:i32)
        n148 = Build Array (concatenate)(w302, w300) -> (w301:dbl[][])
        n149 = case shown="10" w296 {
          selector: w296 -> [w304 _]
          tunnel: w300 -> [_ w308]
          tunnel: w299 -> [w303 w307]
          tunnel: [w303 w306] -> w298
          tunnel: [w304 0] -> w295
          frame 0, Default {
          }
          frame 10 {
            n150 = Enqueue Element(queue=w307, element=w308) -> (queue out=w306:refnum<queue>)  [unwired: 2 in, 2 out]
          }
        }
      }
    }
    n151 = Not Equal To 0?(x=w144) -> (x != 0?=w152:bool)
    n152 = Equal?(x=w145, y=1) -> (x = y?=w153:bool)
    n153 = Or(x=w153, y=w152) -> (x .or. y?=w135:bool)
    n154 = Not(x=w135) -> (.not. x?=w134:bool)
    "finished" <- w134
    n155 = local write "finished"(w134) -> ()
    n156 = global read "ActiveArray.vi" "Active"() -> (w133:bool[])
    n157 = Index Array(array=w133, index=w112) -> (element=w132:bool)
    n158 = Not(x=w132) -> (.not. x?=w131:bool)
    n159 = Or(x="stop 4", y=w131) -> (x .or. y?=w129:bool)
    n160 = case shown="True" w129 {
      tunnel: [w287 w288] -> w149
      tunnel: w139 -> [w287 w289]
      tunnel: w117 -> [_ w291]
      tunnel: w141 -> [_ w290]
      frame False {
      }
      frame True {
        n161 = call "StopChannel.vi"("error in (no error)"=w289, "Channel"=w291, "ID"=w290) -> ("error out"=w288:errorcluster)  [unwired: 8 in]
      }
    }
    n162 = local read "MPP start time"() -> (w122:timestamp)
    n163 = local write "CAData"(w125) -> ()
    n164 = Get Date/Time In Seconds() -> (seconds since 1Jan1904=w120:timestamp)
    n165 = Add(x=w122, y=w121) -> (x+y=w119:timestamp)
    n166 = Greater?(x=w120, y=w119) -> (0:w118:bool)
    n167 = local write "Time has Elapsed"(w118) -> ()
    n168 = Wait Until Next ms Multiple(millisecond multiple=u32 100) -> ()  [unwired: 1 out]
  }
  "error out" <- w31
  n169 = Release Queue(queue=w13) -> ()  [unwired: 2 in, 3 out]
  n170 = Release Queue(queue=w7) -> ()  [unwired: 2 in, 3 out]
  "last time" <- w30
  "Aging Data" <- dbl[][] []
